vi "intializing_using_variable.vi"() -> ()   [LabVIEW 2019]
panel:
  out "Numeric":i32
  in  "stop":bool
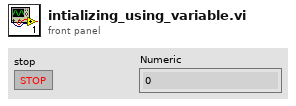
[diagram p1: front panel]
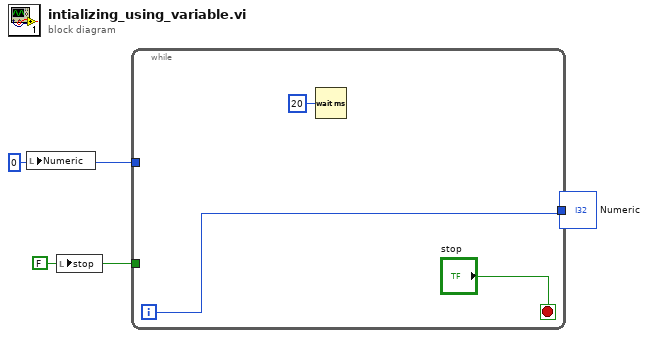
[diagram p0: block diagram]
diagram:
  w1 = FALSE ("stop")
  w2 = 0 ("Numeric")
  n1 = local write "Numeric"(w2) -> ()
  n2 = local write "stop"(w1) -> ()
  n3 = while {
    tunnel: [w5] -> w3
    tunnel: w2 -> [_]
    tunnel: w1 -> [_]
    i -> [w5]
    stop <- "stop" stop-if-true
    n4 = Wait (ms)(milliseconds to wait=u32 20) -> ()  [unwired: 1 out]
  }
  "Numeric" <- w3
